vi "Control Servo.vi"(8 "error in (no error)":errorcluster, 9 "force (V)":dbl, 10 "setpoint (V)":dbl, 11 "PID Controller in":refnum<class "PID Controller.lvclass">) -> (0 "error out":errorcluster, 2 "servo pw (us)":dbl, 3 "PID Controller out":refnum<class "PID Controller.lvclass">)   [LabVIEW 2020, in "PID Controller.lvclass"]
uses:
  PID Controller.lvclass
  C:/Users/jharw/Documents/1 Folder to Rule them All/UMD/Inflation-Apparatus/src/Controllers/Controller.lvclass
  Controller.lvclass/Controller.ctl
  PID Controller.lvclass/PID Controller.ctl
  <vilib>/addons/control/pid/pid.llb/PID (DBL).vi
  <vilib>/addons/control/pid/NI_PID_pid.lvlib
  Controller.lvclass
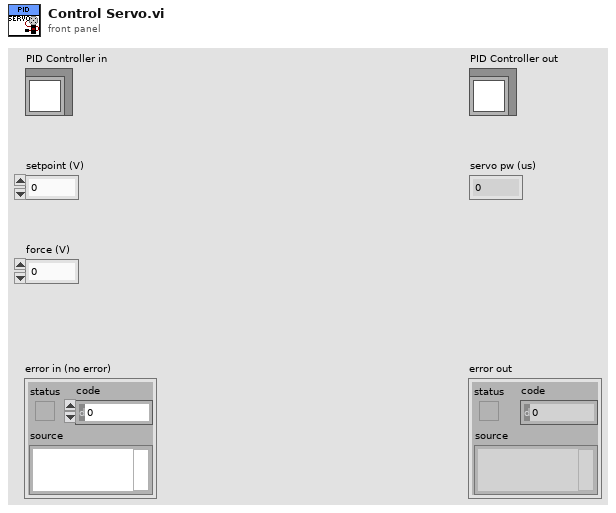
[diagram p1: front panel]
types:
  T1 = cluster{"proportional gain (Kc)":dbl, "integral time (Ti, min)":dbl, "derivative time (Td, min)":dbl}
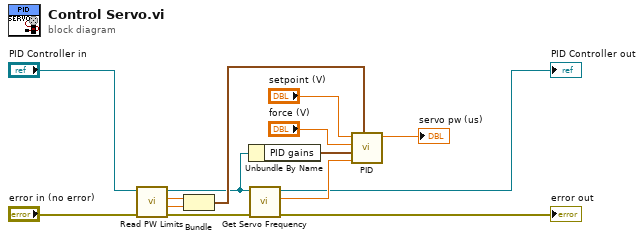
[diagram p0: block diagram]
diagram:
  n1 = call "Read PW Limits.vi"("error in (no error)"="error in (no error)", "Controller in"="PID Controller in") -> ("error out"=w5:errorcluster, "low pw (us)"=w12:dbl, "high pw (us)"=w13:dbl, "Controller out"=w1:refnum<class "PID Controller.lvclass">)  [unwired: 6 in]
  n2 = Bundle("high pw (us)"=w13, "low pw (us)"=w12) -> (w11:cluster{"high pw (us)":dbl, "low pw (us)":dbl})  [unwired: 1 in]
  n3 = Unbundle By Name(w1) -> ("PID gains"=w6:T1)
  n4 = call "Get Servo Frequency.vi"("error in (no error)"=w5, "Controller in"=w1) -> ("error out"=→"error out":errorcluster, "servo dt (sec)"=w4:dbl, "Controller out"=→"PID Controller out":refnum<class "PID Controller.lvclass">)  [unwired: 7 in]
  n5 = call-poly <vilib>:"PID.vi"("output range"=w11, "dt (s)"=w4, "PID gains"=w6, "process variable"="force (V)", "setpoint"="setpoint (V)") -> ("output"=→"servo pw (us)":dbl)  [unwired: 5 in, 1 out]
